vi "poly_asynch_wait_start.vi"(8 "error in":errorcluster, 9 "ignore previous (T)":bool=TRUE, 10 "notifier (create)":T1) -> (0 "error out":errorcluster, 1 "notifier":T1, 2 "asynch wait ref out":T2)   [LabVIEW 2015, in "_timing_tools_polys.lvlib"]
uses:
  _timing_tools_polys.lvlib
  asynch_wait_ref.ctl
  boolean_notifier.ctl
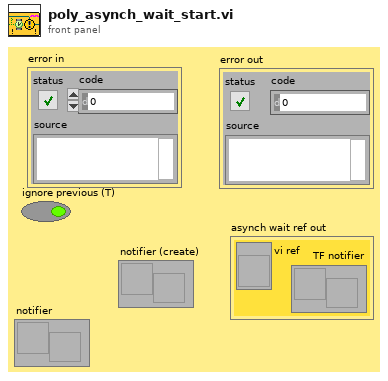
[diagram p1: front panel]
types:
  T1 = typedef "_timing_tools_polys.lvlib/boolean_notifier.ctl" = refnum<notifier>
  T2 = typedef "_timing_tools_polys.lvlib/asynch_wait_ref.ctl" = cluster{"vi ref":refnum<vi>, "TF notifier":T1}
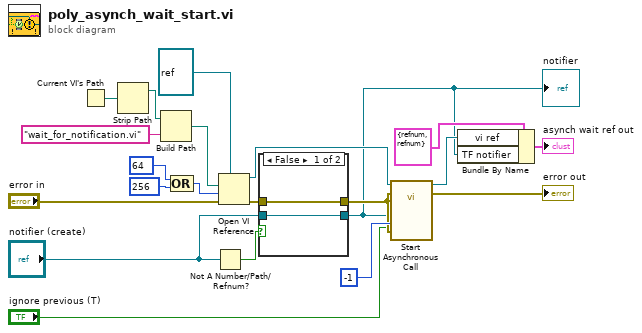
[diagram p0: block diagram]
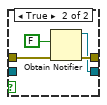
[diagram p2: hidden frame]
diagram:
  n1 = Current VI's Path() -> (path=w21:path)
  n2 = Strip Path(path=w21) -> (stripped path=w20:path)  [unwired: 1 out]
  n3 = Build Path(base path=w20, name or relative path="wait_for_notification.vi") -> (appended path=w18:path)
  n4 = Compound Arithmetic op=OR(64 ("options"), 256 ("options")) -> (w8:i32)
  n5 = Not A Number/Path/Refnum?(number/path/refnum="notifier (create)") -> (NaN/Path/Refnum?=w14:bool)
  n6 = Open VI Reference(type specifier VI Refnum (for type only)=refnum<vi> refnum, vi path=w18, options=w8, error in (no error)="error in") -> (vi reference=w16:refnum<vi>, error out=w6:errorcluster)  [unwired: 2 in]
  n7 = case shown="False" w14 {
    tunnel: "notifier (create)" -> [w23 _]
    tunnel: w6 -> [w22 w27]
    tunnel: [w22 w26] -> w5
    tunnel: [w23 w24] -> w1
    frame False {
    }
    frame True {
      n8 = Obtain Notifier(notification data type=FALSE, error in (no error)=w27) -> (notifier out=w24:refnum<notifier>, error out=w26:errorcluster)  [unwired: 2 in, 1 out]
    }
  }
  "notifier" <- w1
  n9 = call-by-ref "Start Asynchronous Call"(reference=w16, error in=w5, "ignore previous (T)"="ignore previous (T)", "Error in"=w5, "ms timeout (-1)"=-1, "notifier"=w1) -> (reference out=w3:refnum<vi>, error out=→"error out":errorcluster)  [unwired: 4 in, 4 out]
  n10 = Bundle By Name(cluster=T2 {"vi ref"=refnum, "TF notifier"=refnum} ("asynch wait ref out"), "vi ref"=w3, "TF notifier"=w1) -> (→"asynch wait ref out":T2)
